vi "SetProgressState.vi"(8 "error in (no error)":errorcluster, 10 "State (No Progress)":i32(ring) items=["NoProgress"=0, "Indeterminate"=1, "Normal"=2, "Error"=4, "Paused"=8], 11 "Window Handle":refnum<k24>) -> (0 "error out":errorcluster, 3 "dup Window Handle":refnum<k24>)   [LabVIEW 2020, in "Progress Bar.lvclass"]
uses:
  <userlib>/_MGI/User Interface/Progress Bar/Progress Bar.lvclass
  C:/Program Files/National Instruments/LabVIEW 2020/user.lib/_MGI/User Interface/Progress Bar/Windows7 Taskbar API/Windows7Taskbar_LV9.dll
  Windows7Taskbar_LV9.dll
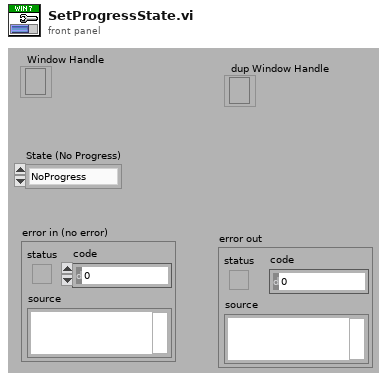
[diagram p1: front panel]
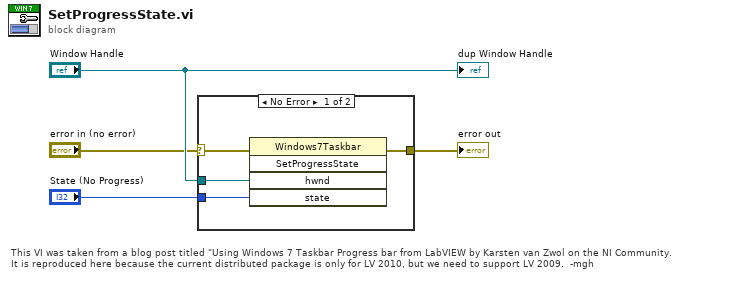
[diagram p0: block diagram]
diagram:
  # "This VI was taken from a blog post titled \"Using Windows 7 Taskbar Progress bar from LabVIEW by Karsten van Zwol on the NI Community.\nIt is reproduced here because the current distributed package is only for LV 2010, but we need to support LV 2009.  -mgh"
  n1 = case shown="No Error" "error in (no error)" {
    selector: "error in (no error)" -> [w5 w9]
    tunnel: [w8 w9] -> w4
    tunnel: "Window Handle" -> [w7 _]
    tunnel: "State (No Progress)" -> [w6 _]
    frame No Error {
      n2 = invoke class="Windows7Taskbar" method="SetProgressState"(error in=w5, "hwnd"=w7, "state"=w6) -> (error out=w8:errorcluster)  [unwired: 2 in, 4 out]
    }
    frame Error {
    }
  }
  "error out" <- w4
  "dup Window Handle" <- "Window Handle"
